vi "test_firmware.vi"() -> ()   [LabVIEW 2025]
doc: "VI para probar que el firmware de LV_ESP32 se haya subido y funcione correctamente"
panel:
  out "read buffer 2":string
  out "WIFI Listo":bool
  in  "START":bool
  out "read buffer":string
  out "ESP32 Listo":bool
  in  "Close":bool
  out "error out":errorcluster
  in  "stop":bool
  in  "Puerto COM":refnum<visa-resource-name>
  # "Este VI es para comprobar si el firmware fue subido correctamente\nSelecciona el puerto en donde este conectada la ESP32 \nLuego presiona el boton START\nEspera unos momentos y veras como comprueba el firmware y la conexion a internet (aun no disponible en feb 2026)\nSi falla la conexion a serial y crees que instalaste bien el firmware presiona el boton RST"
  # "Prueba de Firmware"
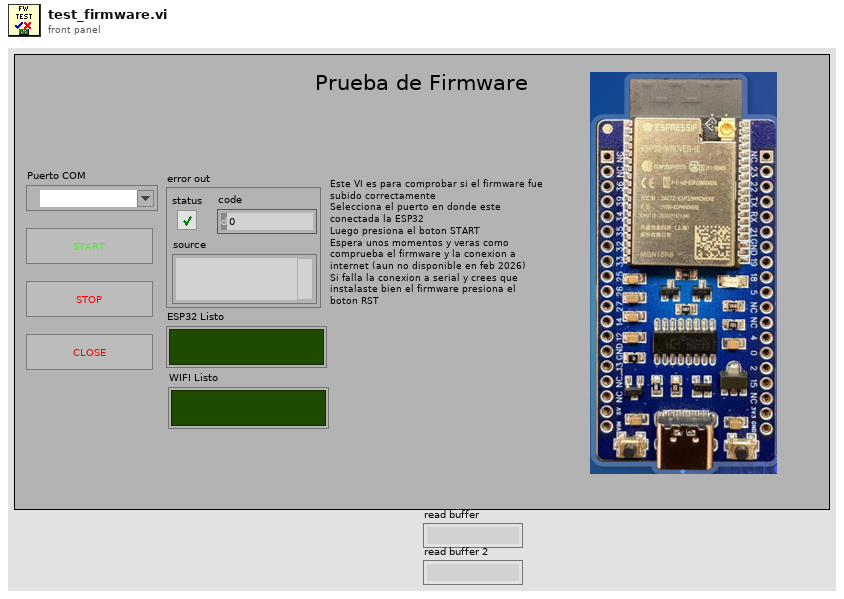
[diagram p1: front panel]
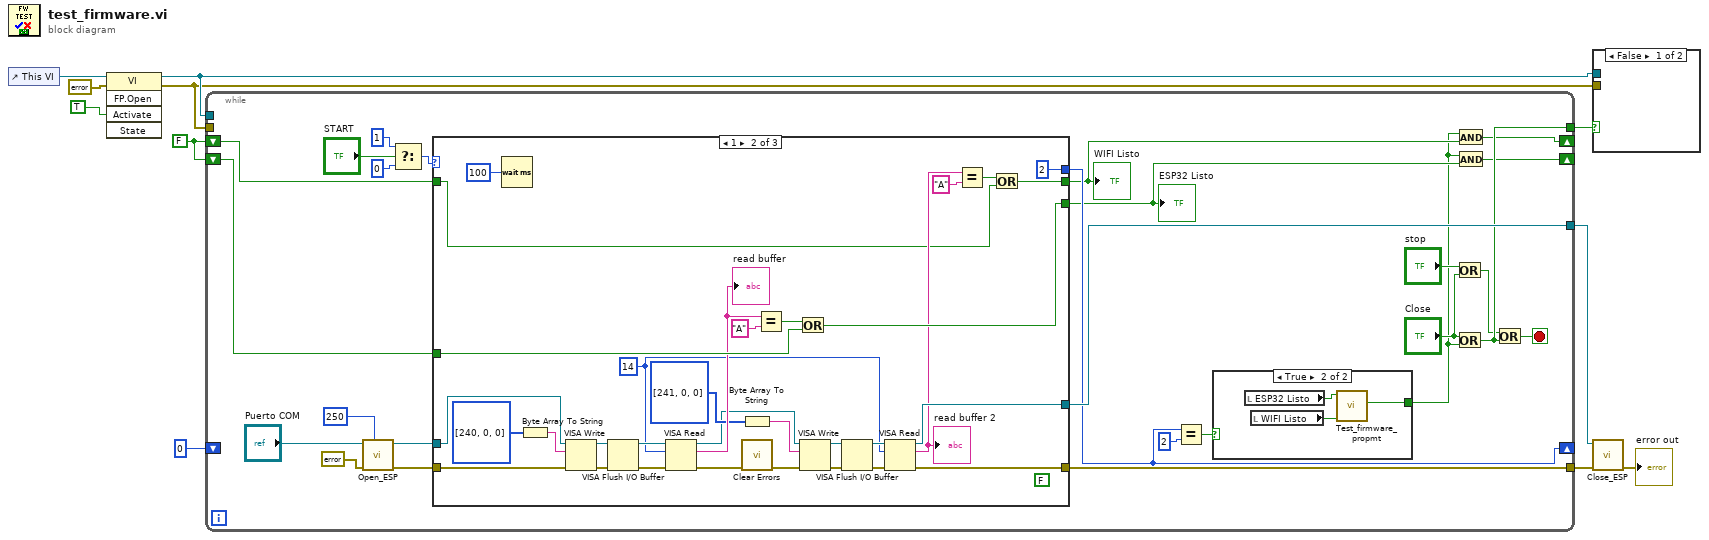
[diagram p0: block diagram]
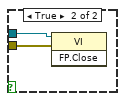
[diagram p2: hidden frame]
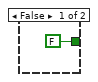
[diagram p3: hidden frame]
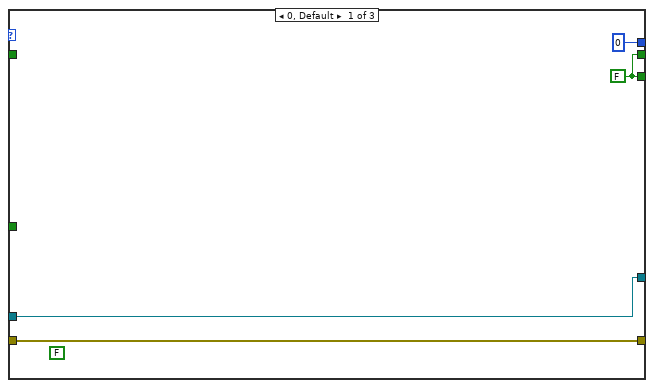
[diagram p4: hidden frame]
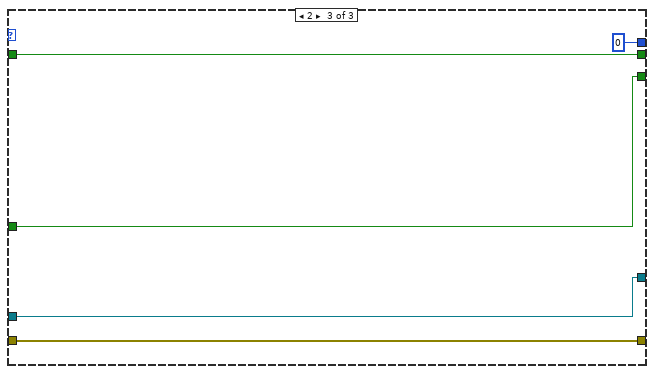
[diagram p5: hidden frame]
diagram:
  w2 = FALSE
  n1 = control-ref of="This VI"() -> (w11:refnum<vi>)
  n2 = invoke class="VI" method="FP.Open"(reference=w11, error in=errorcluster {"status"=FALSE, "code"=0, "source"=""} ("error in (no error)"), "Activate"=TRUE ("Activate?")) -> (reference out=w8:refnum<vi>, error out=w7:errorcluster)  [unwired: 2 in, 3 out]
  n3 = while {
    tunnel: w8 -> [_]
    tunnel: w7 -> [_]
    tunnel: [w27] -> w6
    shift-right: [w21] -> _
    shift-left: w2 -> [w36]
    tunnel: [w35] -> w4
    tunnel: [w34] -> w3
    shift-right: [w20] -> _
    shift-left: w2 -> [w33]
    shift-right: [w23] -> _
    shift-left: u32 0 ("milliseconds to wait") -> [_]
    stop <- w25 stop-if-true
    n4 = call "Open_ESP.vi"("timeout (10sec)"=u32 250, "error in (no error)"=errorcluster {"status"=FALSE, "code"=0, "source"=""}, "VISA resource name"="Puerto COM") -> ("error out"=w13:errorcluster, "VISA resource name out"=w12:refnum<visa-resource-name>)  [unwired: 7 in]
    n5 = Select(t=u32 1 ("milliseconds to wait"), s="START", f=u32 0 ("milliseconds to wait")) -> (s? t:f=w29:u32)
    n6 = case shown="1" w29 {
      tunnel: w36 -> [_ w76 w80]
      tunnel: [w42 w74 w80] -> w18
      tunnel: w13 -> [w44 w72 w82]
      tunnel: w12 -> [w45 w71 w79]
      tunnel: [w44 w70 w82] -> w35
      tunnel: [w45 w69 w79] -> w34
      tunnel: [w42 w65 w78] -> w19
      tunnel: w33 -> [_ w64 w78]
      tunnel: [u32 0 ("milliseconds to wait") u32 2 ("milliseconds to wait") u32 0 ("milliseconds to wait")] -> w23
      frame 0, Default {
        (unwired) FALSE
        w42 = FALSE
      }
      frame 1 {
        (unwired) FALSE
        w50 = u32 14 ("byte count")
        n7 = Wait (ms)(milliseconds to wait=u32 100) -> ()  [unwired: 1 out]
        n8 = Byte Array To String(unsigned byte array=u8[] [240, 0, 0] ("Array")) -> (string=w58:string)
        n9 = VISA Write(VISA resource name=w71, write buffer=w58, error in (no error)=w72) -> (VISA resource name out=w63:refnum<visa-resource-name>, error out=w60:errorcluster)  [unwired: 1 out]
        n10 = VISA Flush I/O Buffer(VISA resource name=w63, error in (no error)=w60) -> (VISA resource name out=w62:refnum<visa-resource-name>, error out=w61:errorcluster)  [unwired: 1 in]
        n11 = VISA Read(VISA resource name=w62, byte count=w50, error in (no error)=w61) -> (VISA resource name out=w51:refnum<visa-resource-name>, read buffer=w68:string, error out=w47:errorcluster)  [unwired: 1 out]
        "read buffer" <- w68
        n12 = Byte Array To String(unsigned byte array=u8[] [241, 0, 0] ("Array")) -> (string=w49:string)
        n13 = call <vilib>:"Clear Errors.vi"("error in (no error)"=w47) -> ("error out"=w48:errorcluster)  [unwired: 5 in, 1 out]
        n14 = Equal?(x=w68, y="A" ("regular expression")) -> (x = y?=w75:bool)
        n15 = Or(x=w75, y=w76) -> (x .or. y?=w74:bool)
        n16 = VISA Write(VISA resource name=w51, write buffer=w49, error in (no error)=w48) -> (VISA resource name out=w53:refnum<visa-resource-name>, error out=w55:errorcluster)  [unwired: 1 out]
        n17 = VISA Flush I/O Buffer(VISA resource name=w53, error in (no error)=w55) -> (VISA resource name out=w52:refnum<visa-resource-name>, error out=w54:errorcluster)  [unwired: 1 in]
        n18 = VISA Read(VISA resource name=w52, byte count=w50, error in (no error)=w54) -> (VISA resource name out=w69:refnum<visa-resource-name>, read buffer=w67:string, error out=w70:errorcluster)  [unwired: 1 out]
        "read buffer 2" <- w67
        n19 = Equal?(x=w67, y="A" ("regular expression")) -> (x = y?=w66:bool)
        n20 = Or(x=w66, y=w64) -> (x .or. y?=w65:bool)
      }
      frame 2 {
      }
    }
    "WIFI Listo" <- w19
    "ESP32 Listo" <- w18
    n21 = Equal?(x=w23, y=u32 2 ("milliseconds to wait")) -> (x = y?=w22:bool)
    n22 = case shown="True" w22 {
      tunnel: [FALSE w39] -> w17
      frame False {
      }
      frame True {
        n23 = local read "ESP32 Listo"() -> (w40:bool)
        n24 = local read "WIFI Listo"() -> (w41:bool)
        n25 = call "Test_firmware_propmt.vi"("WIFI Listo"=w41, "ESP32 Listo"=w40) -> ("Resultado"=w39:bool)  [unwired: 9 in]
      }
    }
    n26 = Or(x="stop", y="Close") -> (x .or. y?=w26:bool)
    n27 = Or(x="Close", y=w17) -> (x .or. y?=w27:bool)
    n28 = And(x=w17, y=w19) -> (x .and. y?=w20:bool)
    n29 = And(x=w17, y=w18) -> (x .and. y?=w21:bool)
    n30 = Or(x=w26, y=w27) -> (x .or. y?=w25:bool)
  }
  n31 = case shown="False" w6 {
    tunnel: w8 -> [_ w84]
    tunnel: w7 -> [_ w83]
    frame False {
    }
    frame True {
      n32 = invoke class="VI" method="FP.Close"(reference=w84, error in=w83) -> ()  [unwired: 1 in, 3 out]
    }
  }
  n33 = call "Close_ESP.vi"("error in (no error)"=w4, "VISA resource name"=w3) -> ("error out"=→"error out":errorcluster)  [unwired: 9 in]
